vi "MtoolTest.vi"() -> ()   [LabVIEW 2019]
panel:
  in  "milliseconds to wait":u32
  out "read buffer":string
  in  "write buffer":string
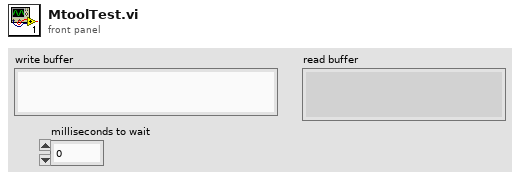
[diagram p1: front panel]
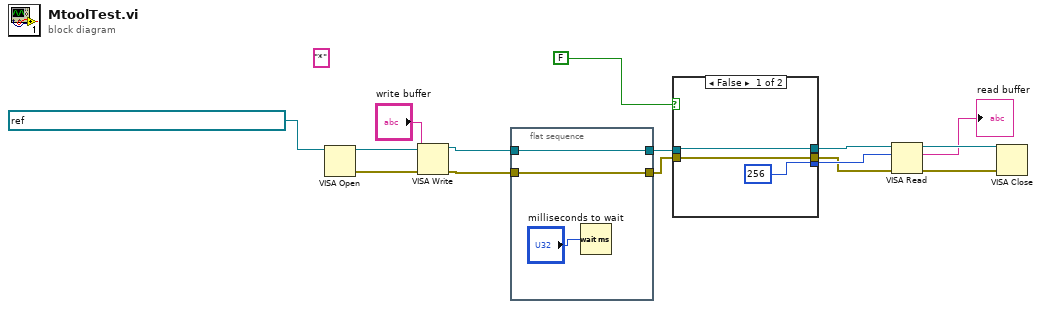
[diagram p0: block diagram]
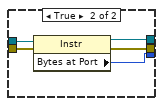
[diagram p2: hidden frame]
diagram:
  (unwired) "*"
  n1 = VISA Open(VISA resource name=refnum<visa-resource-name> "USB0::0x2A8D::0xB318::MY59430005::INSTR") -> (VISA resource name=w15:refnum<visa-resource-name>, error out=w14:errorcluster)  [unwired: 4 in]
  n2 = VISA Write(VISA resource name=w15, write buffer="write buffer", error in (no error)=w14) -> (VISA resource name out=w6:refnum<visa-resource-name>, error out=w10:errorcluster)  [unwired: 1 out]
  n3 = flat-sequence {
    tunnel: w10 -> [w17]
    tunnel: [w17] -> w5
    tunnel: [w16] -> w7
    tunnel: w6 -> [w16]
    frame #0 {
      n4 = Wait (ms)(milliseconds to wait="milliseconds to wait") -> ()  [unwired: 1 out]
    }
  }
  n5 = case shown="False" FALSE ("Boolean") {
    tunnel: [u32 256 ("Bytes at Port") w26] -> w8
    tunnel: w7 -> [w21 w25]
    tunnel: w5 -> [w20 w24]
    tunnel: [w20 w23] -> w4
    tunnel: [w21 w22] -> w3
    frame False {
    }
    frame True {
      n6 = property class="Instr"(reference=w25, error in=w24) -> (reference out=w22:refnum<visa-resource-name>, error out=w23:errorcluster, "Bytes at Port"=w26:u32)
    }
  }
  n7 = VISA Read(VISA resource name=w3, byte count=w8, error in (no error)=w4) -> (VISA resource name out=w12:refnum<visa-resource-name>, read buffer=→"read buffer":string, error out=w11:errorcluster)  [unwired: 1 out]
  n8 = VISA Close(VISA resource name=w12, error in (no error)=w11) -> ()  [unwired: 1 out]
